vi "shift visible array down one.vi"(8 "error in (no error)":errorcluster, 11 "Array in":refnum<vi>) -> (0 "error out":errorcluster, 3 "Array out":refnum<vi>)   [LabVIEW 2015, in "PID Module editor node.lvclass"]
doc: "This VI shifts the array index 1 down to adjust the display"
uses:
  PID Module editor node.lvclass
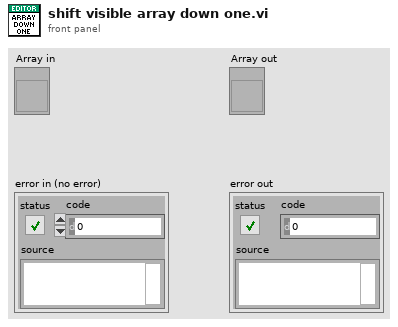
[diagram p1: front panel]
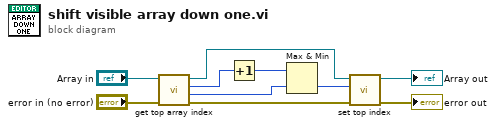
[diagram p0: block diagram]
diagram:
  n1 = call "get top array index.vi"("error in (no error)"="error in (no error)", "Array in"="Array in") -> ("error out"=w2:errorcluster, "last value index"=w1:u32, "top index"=w3:u32, "Array out"=w4:refnum<vi>)  [unwired: 6 in]
  n2 = Increment(x=w3) -> (x+1=w7:u32)
  n3 = Max & Min(x=w7, y=w1) -> (min(x,y)=w8:u32)  [unwired: 1 out]
  n4 = call "set top index.vi"("error in (no error)"=w2, "Numeric"=w8, "Array in"=w4) -> ("error out"=→"error out":errorcluster, "Array out"=→"Array out":refnum<vi>)  [unwired: 7 in]
